vi "Update Intensity Graph.vi"(8 "error in (no error)":errorcluster, 10 "Intensity Graph":u16[][](array[numeric]), 11 "Viewer in":refnum<class "Viewer.lvclass">) -> (0 "error out":errorcluster, 3 "Viewer out":refnum<class "Viewer.lvclass">)   [LabVIEW 2015, in "Viewer.lvlib" / "Viewer.lvclass"]
uses:
  Viewer.lvclass
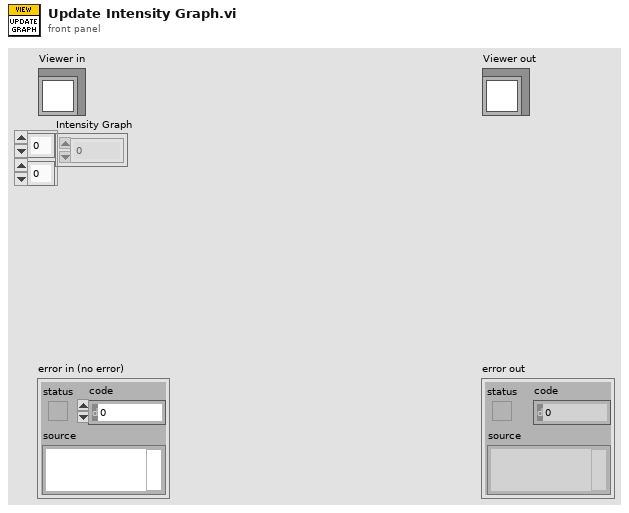
[diagram p1: front panel]
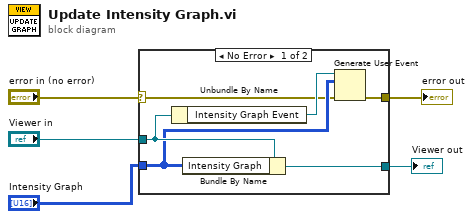
[diagram p0: block diagram]
diagram:
  n1 = case shown="No Error" "error in (no error)" {
    selector: "error in (no error)" -> [w7 w13]
    tunnel: [w6 w13] -> w4
    tunnel: [w11 w12] -> w2
    tunnel: "Viewer in" -> [w10 w12]
    tunnel: "Intensity Graph" -> [w8 _]
    frame No Error {
      n2 = Unbundle By Name(w10) -> ("Intensity Graph Event"=w9:refnum<user-event>)
      n3 = Bundle By Name(cluster=w10, "Intensity Graph"=w8) -> (w11:refnum<class "Viewer.lvclass">)
      n4 = Generate User Event(user event=w9, event data cluster=w8, error in=w7) -> (error out=w6:errorcluster)  [unwired: 1 in, 1 out]
    }
    frame Error {
    }
  }
  "error out" <- w4
  "Viewer out" <- w2
